vi "Set Position.vi"   [LabVIEW 2020, in "video_io.lvlib" / "Reader.lvclass"]
uses:
  Reader.lvclass
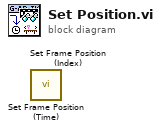
[diagram p0: block diagram]
diagram:
  n1 = call "Set Frame Position (Time).vi"() -> ()  [unwired: 10 in, 2 out]
  n2 = call "Set Frame Position (Index).vi"() -> ()  [unwired: 10 in, 2 out]
